vi "Configure Phase Noise Optimization.vi"(8 "error in (no error)":errorcluster, 10 "Phase Noise Optimization (0: Auto)":i32(ring) items=["Auto", "Fast Tuning", "Best Phase Noise for offsets <20kHz", "Best Phase Noise for offsets >30kHz"], 11 "VISA resource name":refnum<visa-resource-name>) -> (0 "error out":errorcluster, 3 "VISA resource name out":refnum<visa-resource-name>)   [LabVIEW 2014, in "Agilent MXA Series.lvlib"]
doc: "Cofigures the Phase Noize Optimization under List Sweep measurement type."
uses:
  Agilent MXA Series.lvlib
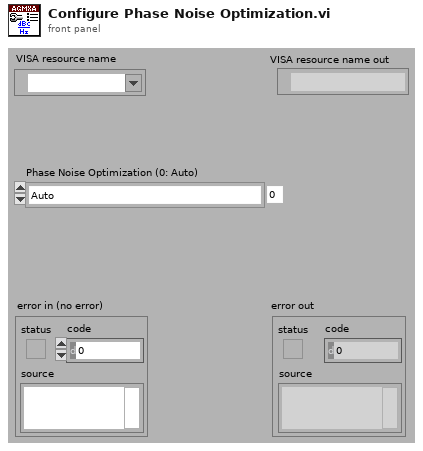
[diagram p1: front panel]
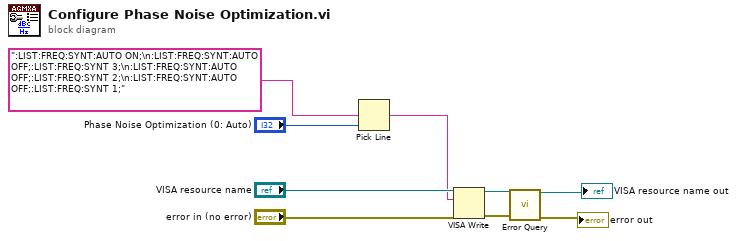
[diagram p0: block diagram]
diagram:
  n1 = Pick Line(multi-line string=":LIST:FREQ:SYNT:AUTO ON;\n:LIST:FREQ:SYNT:AUTO OFF;:LIST:FREQ:SYNT 3;\n:LIST:FREQ:SYNT:AUTO OFF;:LIST:FREQ:SYNT 2;\n:LIST:FREQ:SYNT:AUTO OFF;:LIST:FREQ:SYNT 1;", line index="Phase Noise Optimization (0: Auto)") -> (output string=w1:string)  [unwired: 1 in]
  n2 = VISA Write(VISA resource name="VISA resource name", write buffer=w1, error in (no error)="error in (no error)") -> (VISA resource name out=w6:refnum<visa-resource-name>, error out=w7:errorcluster)  [unwired: 1 out]
  n3 = call "Error Query.vi"("error in (no error)"=w7, "VISA resource name"=w6) -> ("error out"=→"error out":errorcluster, "VISA resource name out"=→"VISA resource name out":refnum<visa-resource-name>)  [unwired: 6 in, 2 out]
